vi "SAP Integration.vi"(8 "error in":errorcluster, 11 "Input Parameters":T2) -> (0 "error out":errorcluster, 3 "Output Parameters":T1)   [LabVIEW 2023]
doc: "Modes : \nMode 1 : Obtaining packing instruction; Required : Mode = 1, Operator = 0043, MaterialCode = 604-003-00-00\nMode 2 : Registering the product serial number - For first serial number : \nRequired : Mode = 2, Same Operator and MaterialCode, SerialNo = 3144369-AA01S251219OK02, PackingInstruction = 1 (1-5 options based on chosen packing instruction), ProductVersion = 1\nMode 2 : For every next device, add also HUNo\nMode 3 : Temporary closed, Required : Mode, Operator, MaterialCode, PackingInstruction and ProductionVersion\nMode 4 : Permanent close, Required : Mode, Operator, MaterialCode, PackingInstruction and ProductionVersion"
uses:
  <userlib>/WebService/_ContactAndRegisterWithNmaSapService/ContactAndRegisterWithNmaSapService.lvlib
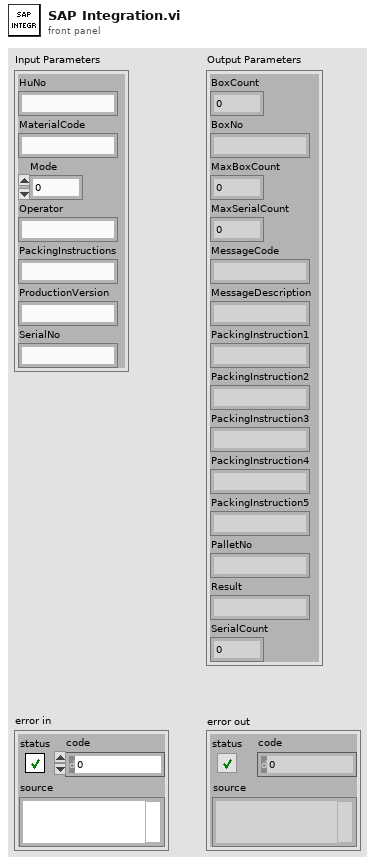
[diagram p1: front panel]
types:
  T1 = cluster{"BoxCount":i32, "BoxNo":string, "MaxBoxCount":i32, "MaxSerialCount":i32, "MessageCode":string, "MessageDescription":string, "PackingInstruction1":string, "PackingInstruction2":string, "PackingInstruction3":string, "PackingInstruction4":string, "PackingInstruction5":string, "PalletNo":string, "Result":string, "SerialCount":i32}
  T2 = cluster{"HuNo":string, "MaterialCode":string, "Mode":i32, "Operator":string, "PackingInstructions":string, "ProductionVersion":string, "SerialNo":string}
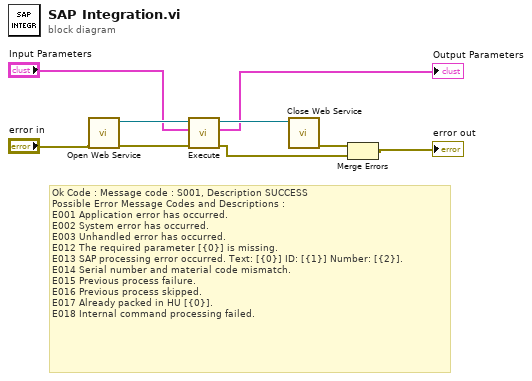
[diagram p0: block diagram]
diagram:
  # "Ok Code : Message code : S001, Description SUCCESS \nPossible Error Message Codes and Descriptions :\nE001 Application error has occurred.\nE002 System error has occurred.\nE003 Unhandled error has occurred.\nE012 The required parameter [{0}] is missing. \nE013 SAP processing error occurred. Text: [{0}] ID: [{1}] Number: [{2}].\nE014 Serial number and material code mismatch.\nE015 Previous process failure.\nE016 Previous process skipped.\nE017 Already packed in HU [{0}].\nE018 Internal command processing failed."
  n1 = call <userlib>:"Open Web Service.vi"("error in (no error)"="error in") -> ("error out"=w8:errorcluster, "ContactAndRegisterWithNmaSapService refnum"=w4:refnum<k24>)  [unwired: 9 in]
  n2 = call <userlib>:"Execute.vi"("error in (no error)"=w8, ".NET:ContactAndRegisterWithNmaSapService.SerialNoRegisterRequest"="Input Parameters", "ContactAndRegisterWithNmaSapService refnum"=w4) -> ("error out"=w6:errorcluster, ".NET:ContactAndRegisterWithNmaSapService.SerialNoRegisterResponse"=→"Output Parameters":T1, "ContactAndRegisterWithNmaSapService refnum out"=w3:refnum<k24>)  [unwired: 6 in]
  n3 = call <userlib>:"Close Web Service.vi"("ContactAndRegisterWithNmaSapService refnum"=w3) -> ("error out"=w7:errorcluster)  [unwired: 10 in]
  n4 = Merge Errors(w7, w6) -> (→"error out":errorcluster)
